vi "Create timing data.vi"(8 "Interpoints \ninterval (ms)":dbl=100.0, 9 "Total time per point (s)":dbl, 10 "Number of points":i32=3, 11 "Repeat \neach point":i32=1 min=0) -> (3 "localTimeData":timestamp[][](array[timestamp])=[[timestamp(3337676887.8125 s since 1904-01-01), timestamp(3337686971.8125 s since 1904-01-01), timestamp(3337697055.8125 s since 1904-01-01)]])   [LabVIEW 2013, in "Phosphorescence - Mode.lvlib"]
uses:
  Phosphorescence - Mode.lvlib
panel:
  out "Time array":dbl[](array[numeric])
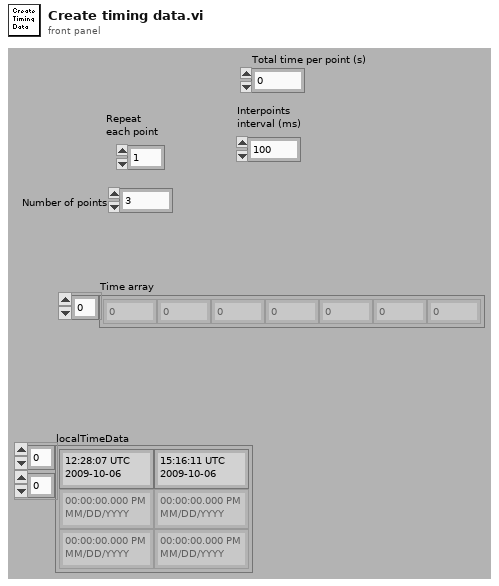
[diagram p1: front panel]
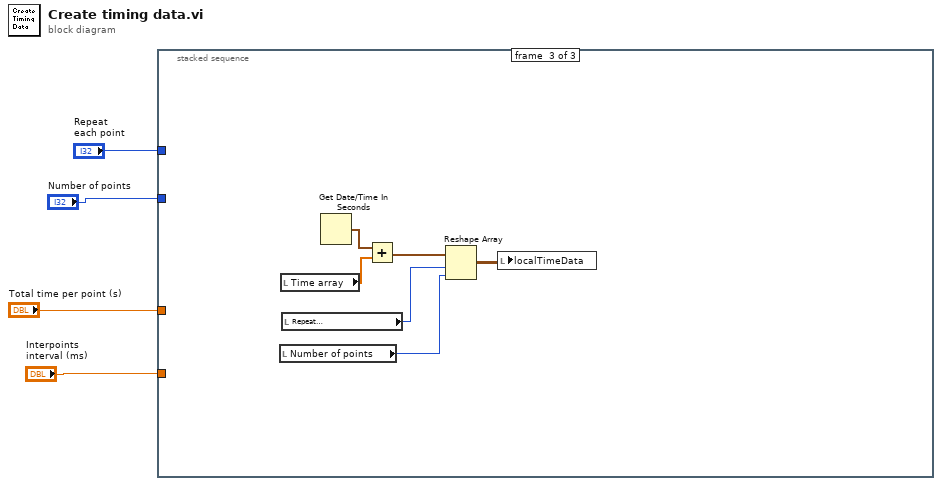
[diagram p0: block diagram]
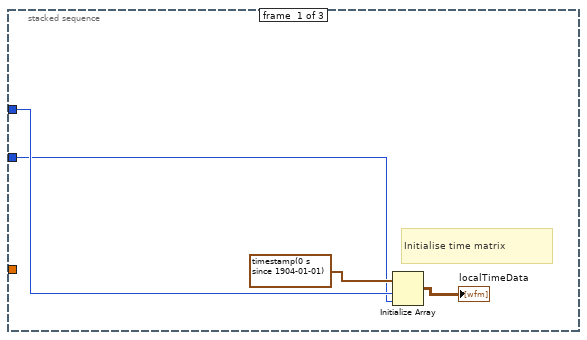
[diagram p2: hidden frame]
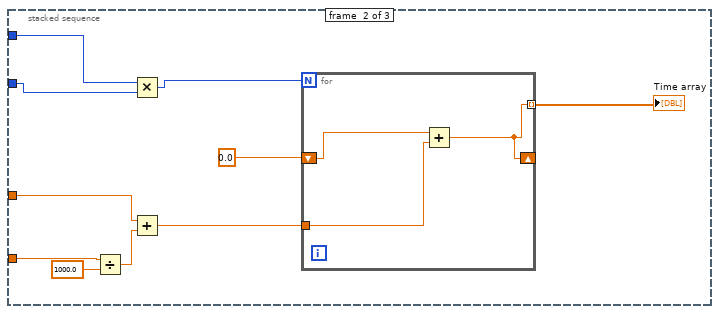
[diagram p3: hidden frame]
diagram:
  n1 = stacked-sequence {
    tunnel: "Number of points" -> [w5 w10 _]
    tunnel: "Repeat \neach point" -> [w7 w11 _]
    tunnel: "Interpoints \ninterval (ms)" -> [_ w18 _]
    tunnel: "Total time per point (s)" -> [_ w16 _]
    frame #0 {
      # "Initialise time matrix"
      n2 = Initialize Array(timestamp(0 s since 1904-01-01) ("temps actuel"), w7, w5) -> (→"localTimeData":timestamp[][])
    }
    frame #1 {
      n3 = Divide(x=w18, y=1000.0) -> (x/y=w15:dbl)
      n4 = Multiply(x=w11, y=w10) -> (x*y=w9:i32)
      n5 = Add(x=w16, y=w15) -> (x+y=w14:dbl)
      n6 = for {
        N: w9 -> [_]
        shift-right: [w19] -> _
        shift-left: 0.0 ("y") -> [w21]
        tunnel: w14 -> [w20]
        tunnel: [w19] -> w12 mode=indexing
        n7 = Add(x=w21, y=w20) -> (x+y=w19:dbl)
      }
      "Time array" <- w12
    }
    frame #2 {
      n8 = local read "Number of points"() -> (w23:i32)
      n9 = local read "Time array"() -> (w26:dbl[])
      n10 = local read "Repeat \neach point"() -> (w24:i32)
      n11 = Get Date/Time In Seconds() -> (seconds since 1Jan1904=w27:timestamp)
      n12 = Add(x=w27, y=w26) -> (x+y=w25:timestamp[])
      n13 = Reshape Array(w25, w24, w23) -> (w22:timestamp[][])
      n14 = local write "localTimeData"(w22) -> ()
    }
  }
